vi "(Sub_VI)_Control_tabs_AOs_reset.vi"(0 "task in":refnum<k21>, 2 "Package for PID":T1, 3 "physical channels":tag, 5 "error in":errorcluster) -> (6 "task out":refnum<k21>, 8 "error out":errorcluster)   [LabVIEW 2012]
doc: "I. Description:\nThis example demonstrates how to continuously output a waveform using an internal sample clock. The automatic regeneration of data has been disabled, so new data has to be provided throughout the duration of the continuous Analog Output operation. This allows the generation of any arbitrary frequency as this VI computes new data for each iteration of the loop, maintaining phase continuity of the signal. The regeneration of data has also been adjusted so that the newest data is output as quickly as possible; thus reducing the lag between the changing of the data and the output of that data.\n\nII. Instructions for Running:\n1. Select the Physical Channel to correspond to where your signal is output on the DAQ device.\n2. Enter the Minimum and Maximum Voltage range.\n3. Specify the desired Sample Clock Rate of the output Waveform. Higher sample clock rates will produce a smoother waveform.\n4. Manually specify the Analog Output buffer size, in number of samples. A larger buffer would help non-regenerative operations avoid errors due to occasional high CPU load. \nNote: \nThe Analog Output buffer has to be at least as big as the amount of data being written to the board per iteration. The recommended buffer size would be at least twice the amount of data being written to the board per iteration.\n5. Enter the Waveform Information. See the documentation of the Basic Function Generator SubVI for information on each parameter.\n\nIII. Block Diagram Steps:\n1. Create an Analog Output Voltage channel.\n2. Configure the task to prohibit the automatic regeneration of data.\n2a. Set the transfer condition to Less than Full. Allows for more rapid updates of Output Buffer.\n3. Call the DAQmx (Sample Clock) VI to set the sample clock rate. Additionally, set the sample mode to Continuous.\n4. Read the actual sample clock rate (eventually coerced depending on the hardware used). \n5. Compute the desired waveform, using the buffer size and the actual update rate. This VI keeps track of the phase of the waveform to ensure that the generated signal is continuous.\n6. Write the waveform to the output buffer. \n7a. Call the Start VI. This is only needed when the loop is executed for the first time.\n7b. Do nothing.\n8. Loop continuously until user presses the Stop button. Every iteration computes and writes a new waveform to the buffer.\n9. Call the Clear Task VI to clear the Task.\n10. Use the popup dialog box to display an error or warning if any.\n\nIV. I/O Connections Overview:\nMake sure your signal output terminal matches the Physical Channel I/O Control. For further connection information, refer to your hardware reference manual."
uses:
  <vilib>/DAQmx/write.llb/DAQmx Write (Analog 2D DBL NChan NSamp).vi
  <vilib>/DAQmx/create/channels.llb/DAQmx Create Channel (AO-Voltage-Basic).vi
  <vilib>/DAQmx/miscellaneous.llb/DAQmx Fill In Error Info.vi
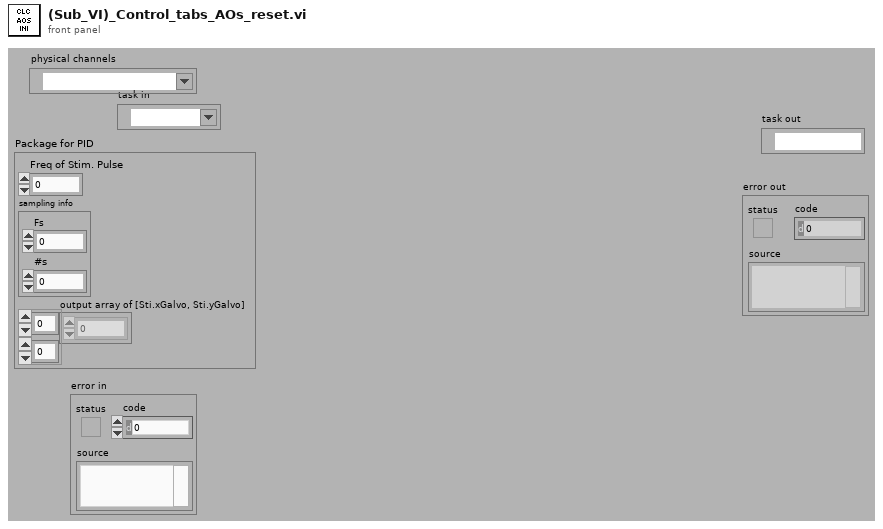
[diagram p1: front panel]
types:
  T1 = cluster{"Freq of Stim. Pulse":dbl, "sampling info":cluster{"Fs":dbl, "#s":dbl}, "output array of [Sti.xGalvo, Sti.yGalvo]":dbl[][]}
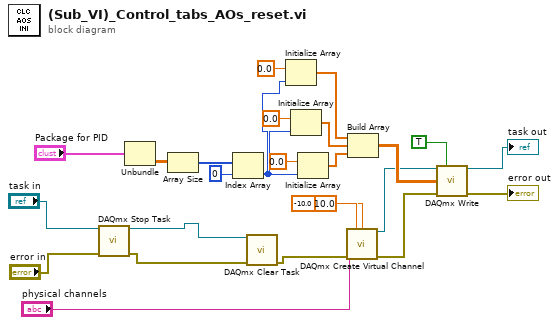
[diagram p0: block diagram]
diagram:
  n1 = call <vilib>:"DAQmx Stop Task.vi"("task/channels in"="task in", "error in"="error in") -> ("task out"=w8:refnum<k21>, "error out"=w7:errorcluster)  [unwired: 12 in]
  n2 = Unbundle("Package for PID") -> ("output array of [Sti.xGalvo, Sti.yGalvo]"=w19:dbl[][])  [unwired: 2 out]
  n3 = Array Size(array=w19) -> (size(s)=w25:i32[])
  n4 = Index Array(array=w25, index=0) -> (element=w13:i32)
  n5 = call <vilib>:"DAQmx Clear Task.vi"("task in"=w8, "error in"=w7) -> ("error out"=w6:errorcluster)  [unwired: 13 in]
  n6 = Initialize Array(0.0 ("element"), w13) -> (w11:dbl[])
  n7 = Initialize Array(0.0 ("element"), w13) -> (w12:dbl[])
  n8 = Initialize Array(0.0 ("element"), w13) -> (w21:dbl[])
  n9 = call-poly <vilib>:"DAQmx Create Virtual Channel.vi"("maximum value"=10.0, "minimum value"=-10.0, "physical channels"="physical channels", "error in"=w6) -> ("task out"=w3:refnum<k21>, "error out"=w2:errorcluster)  [unwired: 10 in]
  n10 = Build Array(w11, w12, w21) -> (w20:dbl[][])
  n11 = call-poly <vilib>:"DAQmx Write.vi"("task/channels in"=w3, "auto start"=TRUE, "data"=w20, "error in"=w2) -> ("task out"=→"task out":refnum<k21>, "error out"=→"error out":errorcluster)  [unwired: 9 in, 1 out]
